vi "setNewItem.vi"(0 "reference in":refnum<class "checkOUT.lvclass">, 2 "index":i32, 3 "dim":i32, 5 "error in (no error)":errorcluster) -> (14 "reference out":refnum<class "checkOUT.lvclass">, 19 "error out":errorcluster)   [LabVIEW 2014, in "checkOUT.lvclass"]
uses:
  checkOUT.lvclass
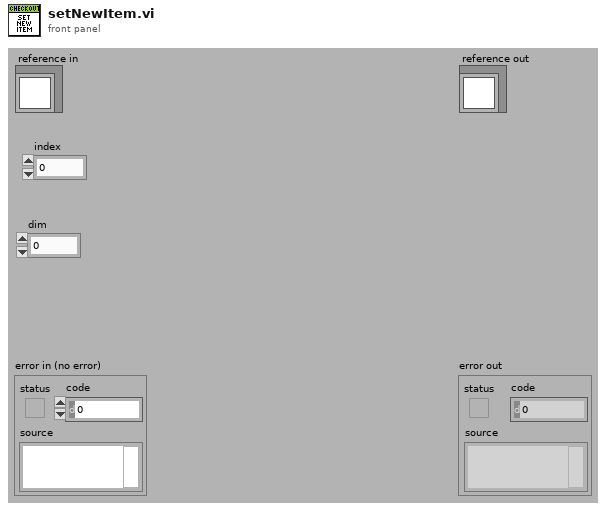
[diagram p1: front panel]
types:
  T1 = typedef "checkOUT.lvclass/ObjectAttributesRef.ctl" = refnum<data-value>
  T2 = typedef "checkOUT.lvclass/ObjectAttributes.ctl" = cluster{"MyAttribute":dbl, "data":string[][]}
  T3 = typedef "checkOUT.lvclass/ClassAttributesRef.ctl" = refnum<data-value>
  T4 = typedef "checkOUT.lvclass/ClassAttributes.ctl" = cluster{"Dummy":bool, "product_refs":refnum<class "checkOUT.lvclass">[]}
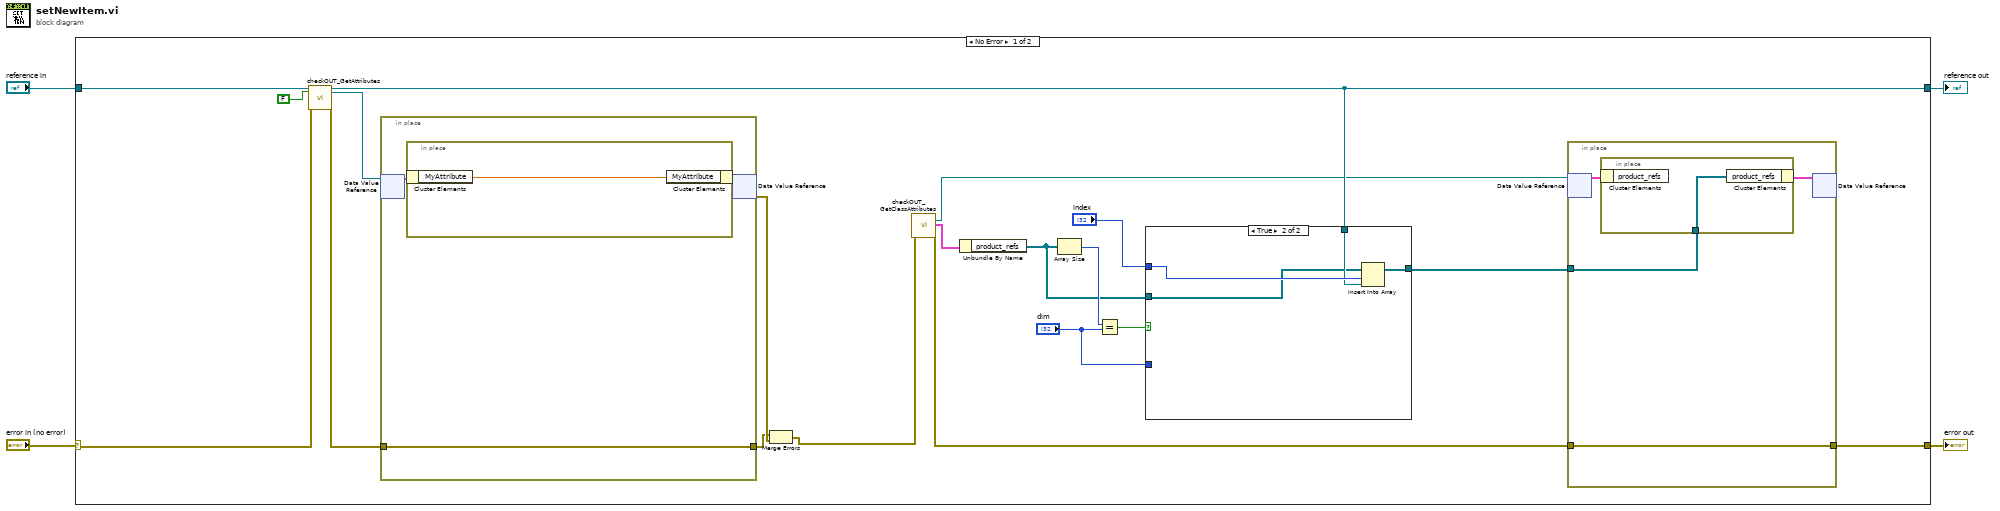
[diagram p0: block diagram]
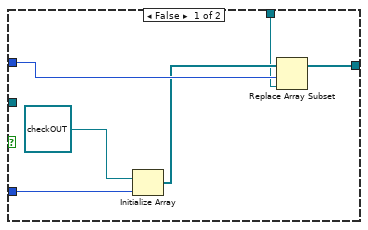
[diagram p2: hidden frame]
diagram:
  n1 = case shown="No Error" "error in (no error)" {
    selector: "error in (no error)" -> [w19 w44]
    tunnel: [w11 w44] -> w3
    tunnel: [w13 w43] -> w1
    tunnel: "reference in" -> [w21 w43]
    frame No Error {
      n2 = call "checkOUT_GetAttributes.vi"("reference in"=w21, "return data? (T)"=FALSE, "error in (no error)"=w19) -> ("reference out"=w13:refnum<class "checkOUT.lvclass">, "attributes ref"=w17:T1, "error out"=w18:errorcluster)  [unwired: 13 in, 1 out]
      n3 = in-place {
        in-place-border: w18 -> [w39]
        in-place-border: [w39] -> w22
        n4 = in-place-dvr #1(w17) -> (w40:T2)  [unwired: 1 out]
        n5 = in-place {
          n6 = in-place-cluster #2(w40) -> ("MyAttribute"=w42:dbl)
          n7 = in-place-cluster #2("MyAttribute"=w42) -> (w41:T2)
        }
        n8 = in-place-dvr #1(w41) -> (w23:errorcluster)  [unwired: 1 out]
      }
      n9 = Merge Errors(w22, w23) -> (w8:errorcluster)
      n10 = call "checkOUT_GetClassAttributes.vi"("error in (no error)"=w8) -> ("class attributes ref"=w10:T3, "class attributes"=w16:T4, "error out"=w12:errorcluster)  [unwired: 15 in, 1 out]
      n11 = Unbundle By Name(w16) -> ("product_refs"=w5:refnum<class "checkOUT.lvclass">[])
      n12 = Array Size(array=w5) -> (size(s)=w15:i32)
      n13 = Equal?(x=w15, y="dim") -> (x = y?=w14:bool)
      n14 = case shown="True" w14 {
        tunnel: "index" -> [w34 w38]
        tunnel: w13 -> [w29 w37]
        tunnel: [w32 w36] -> w9
        tunnel: "dim" -> [w31 _]
        tunnel: w5 -> [_ w35]
        frame False {
          n15 = Initialize Array(refnum<class "checkOUT.lvclass"> refnum ("product.lvclass"), w31) -> (w33:refnum<class "checkOUT.lvclass">[])
          n16 = Replace Array Subset(array=w33, new element=w29, index=w34) -> (w32:refnum<class "checkOUT.lvclass">[])
        }
        frame True {
          n17 = Insert Into Array(array=w35, index=w38, new element=w37) -> (w36:refnum<class "checkOUT.lvclass">[])
        }
      }
      n18 = in-place {
        in-place-border: w12 -> [w25]
        in-place-border: [w25] -> w11
        in-place-border: w9 -> [w24]
        n19 = in-place-dvr #3(w10) -> (w26:T4)  [unwired: 1 out]
        n20 = in-place {
          in-place-border: w24 -> [w28]
          n21 = in-place-cluster #4(w26) -> ()  [unwired: 1 out]
          n22 = in-place-cluster #4("product_refs"=w28) -> (w27:T4)
        }
        n23 = in-place-dvr #3(w27) -> ()  [unwired: 2 out]
      }
    }
    frame Error {
    }
  }
  "error out" <- w3
  "reference out" <- w1
